vi "get_length.vi"(8 "error in (no error)":errorcluster, 11 "DataFrame in":refnum<class "DataFrame.lvclass">) -> (0 "error out":errorcluster, 2 "length":u32, 3 "DataFrame out":refnum<class "DataFrame.lvclass">)   [LabVIEW 2017]
uses:
  DataFrame.lvclass
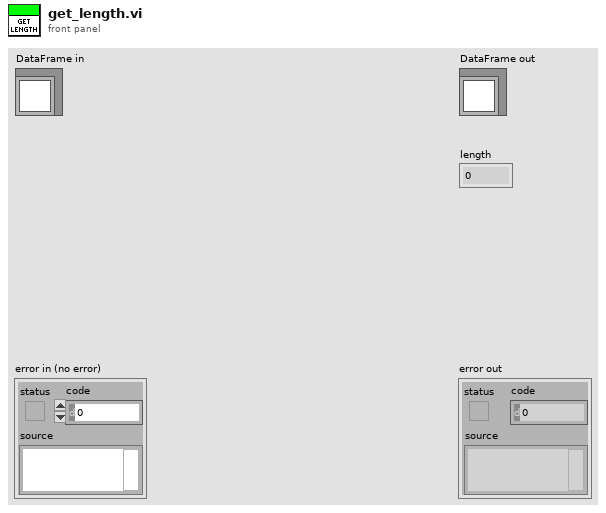
[diagram p1: front panel]
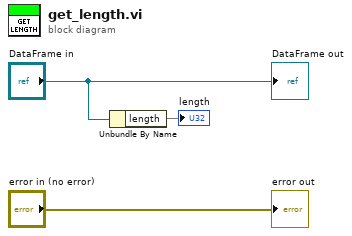
[diagram p0: block diagram]
diagram:
  n1 = Unbundle By Name("DataFrame in") -> ("length"=→"length")
  "error out" <- "error in (no error)"
  "DataFrame out" <- "DataFrame in"
